vi "Check Barcode Required Parameter.vi"(8 "ErrorIn":errorcluster, 11 "VISAIn":refnum<visa-resource-name>) -> (0 "ErrorOut":errorcluster, 2 "Yes?":bool, 3 "VISAOut":refnum<visa-resource-name>)   [LabVIEW 2017, in "I28Drivers.lvlib"]
uses:
  I28Drivers.lvlib
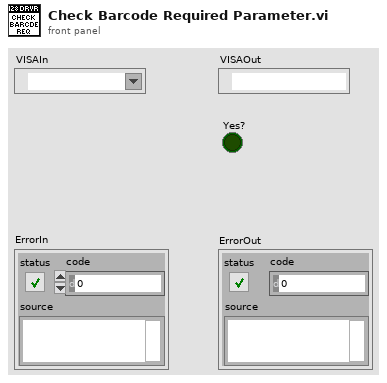
[diagram p1: front panel]
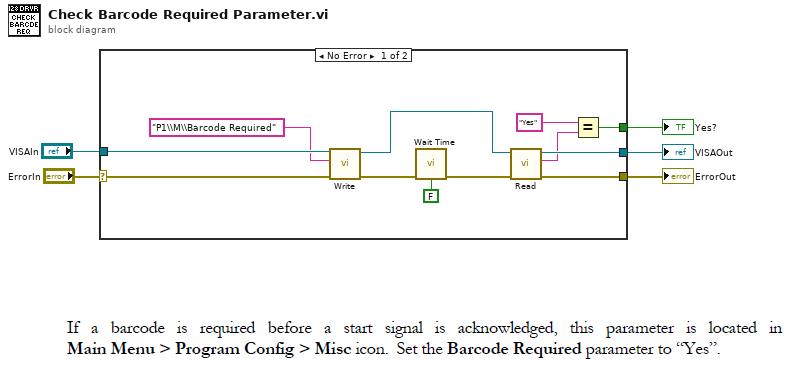
[diagram p0: block diagram]
diagram:
  n1 = case shown="No Error" "ErrorIn" {
    selector: "ErrorIn" -> [w17 w19]
    tunnel: "VISAIn" -> [w16 w18]
    tunnel: [w15 w19] -> w3
    tunnel: [w14 w18] -> w2
    tunnel: [w10 _] -> w1
    frame No Error {
      n2 = call "Write.vi"("ErrorIn"=w17, "Command"="P1\\M\\Barcode Required" ("string"), "VISAIn"=w16) -> ("ErrorOut"=w8:errorcluster, "VISAOut"=w9:refnum<visa-resource-name>)  [unwired: 7 in]
      n3 = call "Wait Time.vi"("error in"=w8, "Set Time"=FALSE) -> ("error out"=w7:errorcluster)  [unwired: 13 in]
      n4 = call "Read.vi"("ErrorIn"=w7, "VISAIn"=w9) -> ("ErrorOut"=w15:errorcluster, "Data"=w12:string, "VISAOut"=w14:refnum<visa-resource-name>)  [unwired: 7 in]
      n5 = Equal?(x="Yes", y=w12) -> (x = y?=w10:bool)
    }
    frame Error {
    }
  }
  "ErrorOut" <- w3
  "VISAOut" <- w2
  "Yes?" <- w1
